vi "GDS_MO_SetEnergy180122.vi"(11 "AEnergy":dbl=8.0) -> ()   [LabVIEW 2015]
uses:
  <userlib>/caLab/Private/Get_PV.vi
  <userlib>/caLab/Private/Put_I32_PV.vi
  <userlib>/caLab/Private/Put_DBL_PV.vi
  <userlib>/caLab/Private/Put_I8_PV.vi
panel:
  out "SPEC:BUSY #2":dbl
  out "SPEC:BUSY":dbl
  out "SPEC:INC":dbl
  out "retrun value":i32
  # "SetEnergy"
  # "EPICS"
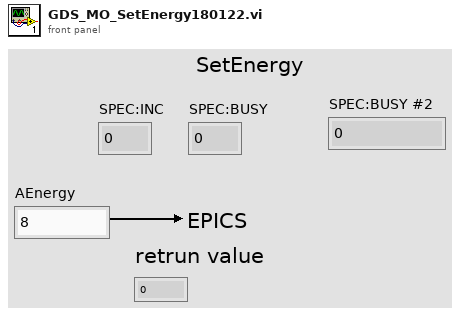
[diagram p1: front panel]
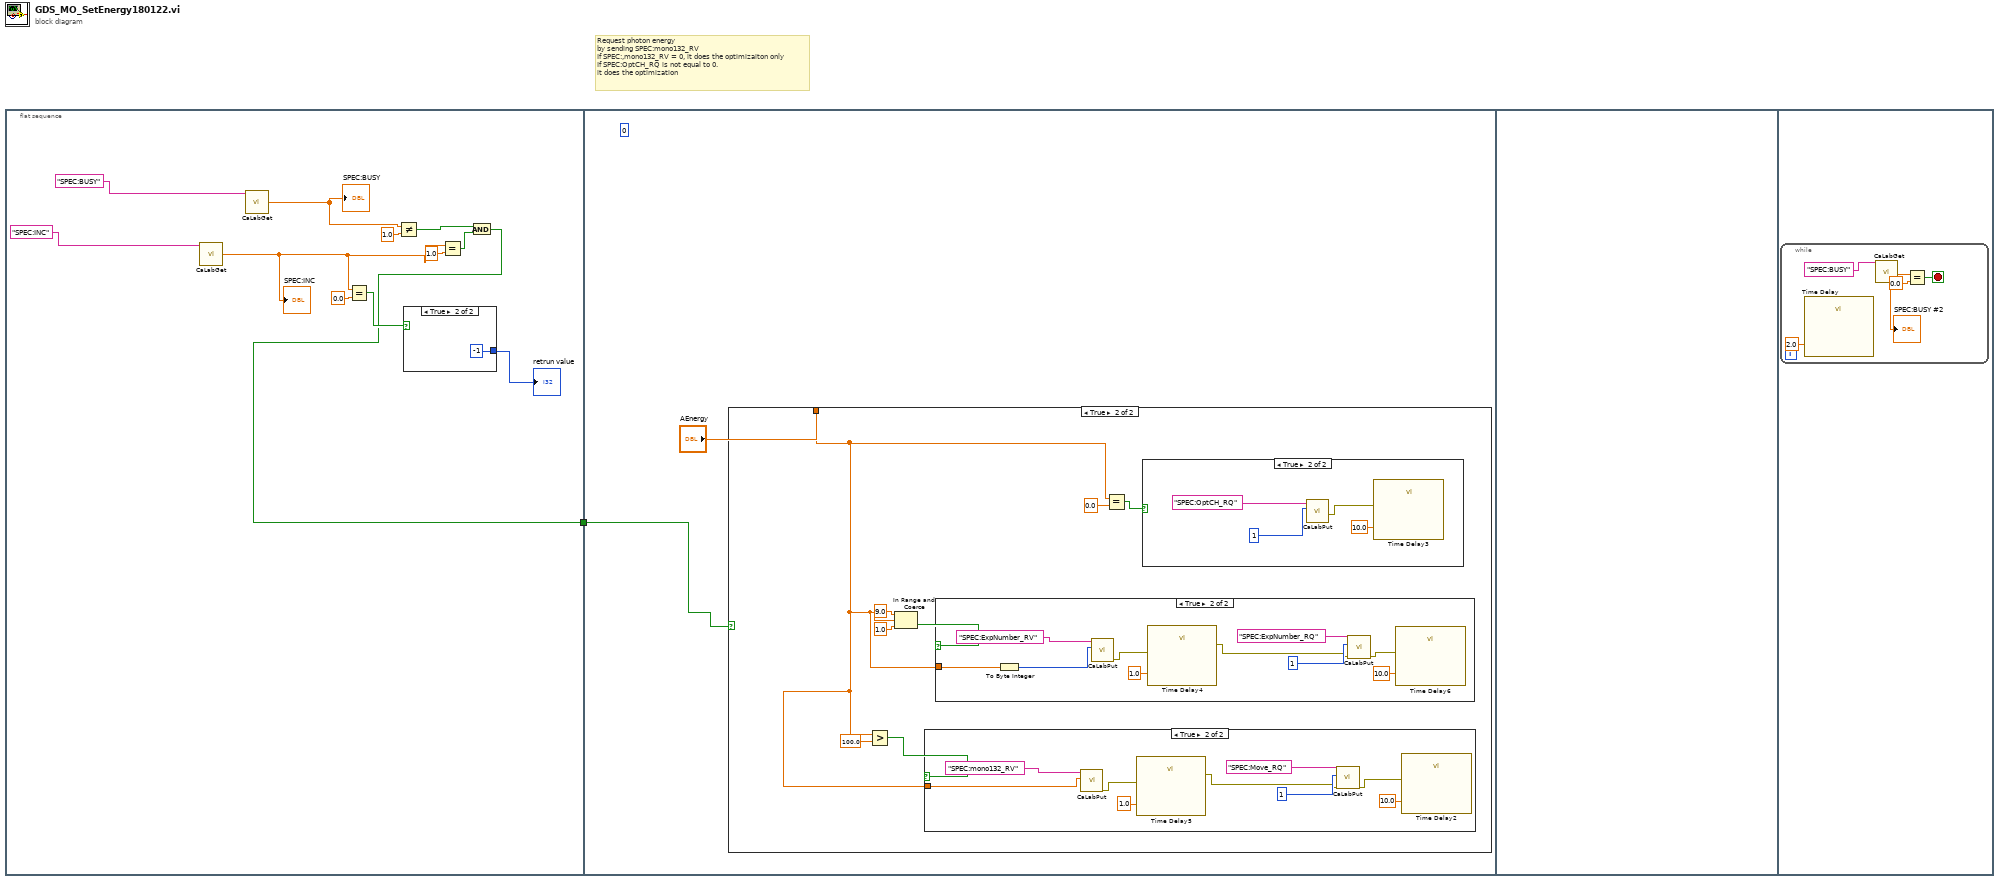
[diagram p0: block diagram]
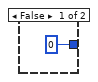
[diagram p2: hidden frame]
diagram:
  # "Request photon energy \nby sending SPEC:mono132_RV\nIf SPEC:,mono132_RV = 0, it does the optimizaiton only\nIf SPEC:OptCH_RQ is not equal to 0.\nit does the optimization"
  n1 = flat-sequence {
    tunnel: [w4] -> w1
    tunnel: w1 -> [w16]
    frame #0 {
      n2 = call-poly <userlib>:"CaLabGet.vi"("PV Name"="SPEC:INC") -> ("1rst Value (number)"=w13:dbl)  [unwired: 8 in, 6 out]
      "SPEC:INC" <- w13
      n3 = call-poly <userlib>:"CaLabGet.vi"("PV Name"="SPEC:BUSY") -> ("1rst Value (number)"=w3:dbl)  [unwired: 8 in, 6 out]
      "SPEC:BUSY" <- w3
      n4 = Equal?(x=w13, y=0.0) -> (x = y?=w6:bool)
      n5 = Not Equal?(x=w3, y=1.0) -> (x != y?=w11:bool)
      n6 = case shown="True" w6 {
        tunnel: [0 -1] -> w7
        frame False {
        }
        frame True {
        }
      }
      "retrun value" <- w7
      n7 = Equal?(x=w13, y=1.0) -> (x = y?=w10:bool)
      n8 = And(x=w11, y=w10) -> (x .and. y?=w4:bool)
    }
    frame #1 {
      (unwired) 0 ("disabled index (col)")
      n9 = case shown="True" w16 {
        tunnel: "AEnergy" -> [_ w18]
        frame False {
        }
        frame True {
          n10 = Greater?(x=w18, y=100.0) -> (0:w20:bool)
          n11 = In Range and Coerce(upper limit=9.0, x=w18, lower limit=1.0) -> (In Range?=w21:bool)  [unwired: 1 out]
          n12 = case shown="True" w20 {
            tunnel: w18 -> [_ w28]
            frame False {
            }
            frame True {
              n13 = call-poly <userlib>:"CaLabPut.vi"("Value"=w28, "PV Name"="SPEC:mono132_RV") -> ("Error out"=w30:errorcluster)  [unwired: 6 in, 3 out]
              n14 = call "Time Delay5"("error in (no error)"=w30, "Delay Time (s)"=1.0) -> ("error out"=w29:errorcluster)  [unwired: 9 in]
              n15 = call-poly <userlib>:"CaLabPut.vi"("Error in (no error)"=w29, "Value"=1, "PV Name"="SPEC:Move_RQ") -> ("Error out"=w26:errorcluster)  [unwired: 5 in, 3 out]
              n16 = call "Time Delay2"("error in (no error)"=w26, "Delay Time (s)"=10.0) -> ()  [unwired: 9 in, 1 out]
            }
          }
          n17 = case shown="True" w21 {
            tunnel: w18 -> [_ w43]
            frame False {
            }
            frame True {
              n18 = To Byte Integer(number=w43) -> (8bit integer=w42:i8)
              n19 = call-poly <userlib>:"CaLabPut.vi"("Value"=w42, "PV Name"="SPEC:ExpNumber_RV") -> ("Error out"=w38:errorcluster)  [unwired: 6 in, 3 out]
              n20 = call "Time Delay4"("error in (no error)"=w38, "Delay Time (s)"=1.0) -> ("error out"=w37:errorcluster)  [unwired: 9 in]
              n21 = call-poly <userlib>:"CaLabPut.vi"("Error in (no error)"=w37, "Value"=1, "PV Name"="SPEC:ExpNumber_RQ") -> ("Error out"=w35:errorcluster)  [unwired: 5 in, 3 out]
              n22 = call "Time Delay6"("error in (no error)"=w35, "Delay Time (s)"=10.0) -> ()  [unwired: 9 in, 1 out]
            }
          }
          n23 = Equal?(x=w18, y=0.0) -> (x = y?=w25:bool)
          n24 = case shown="True" w25 {
            frame False {
            }
            frame True {
              n25 = call-poly <userlib>:"CaLabPut.vi"("Value"=1, "PV Name"="SPEC:OptCH_RQ") -> ("PV error"=w45:errorcluster)  [unwired: 6 in, 3 out]
              n26 = call "Time Delay3"("error in (no error)"=w45, "Delay Time (s)"=10.0) -> ()  [unwired: 9 in, 1 out]
            }
          }
        }
      }
    }
    frame #2 {
    }
    frame #3 {
      n27 = while {
        stop <- w53 stop-if-true
        n28 = call "Time Delay"("Delay Time (s)"=2.0) -> ()  [unwired: 10 in, 1 out]
        n29 = call-poly <userlib>:"CaLabGet.vi"("PV Name"="SPEC:BUSY") -> ("1rst Value (number)"=w51:dbl)  [unwired: 8 in, 6 out]
        "SPEC:BUSY #2" <- w51
        n30 = Equal?(x=w51, y=0.0) -> (x = y?=w53:bool)
      }
    }
  }
